vi "Page_Source_Send_To_MainDest_OnAdd.vi"(8 "error in (no error)":errorcluster, 11 "AB_Targetfile in":refnum<class "AB_Targetfile.lvclass">) -> (0 "error out":errorcluster, 2 "send to main dest":bool, 3 "AB_Targetfile out":refnum<class "AB_Targetfile.lvclass">)   [LabVIEW 2020, in "AB_Targetfile.lvclass"]
uses:
  <vilib>/AppBuilder/AB_Classes/TargetFile/AB_Targetfile.lvclass
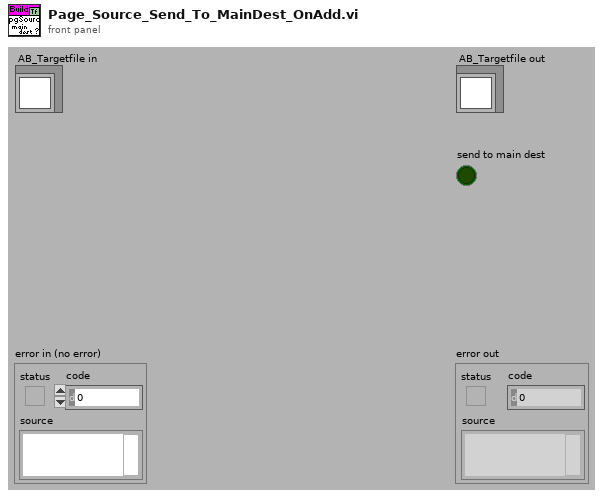
[diagram p1: front panel]
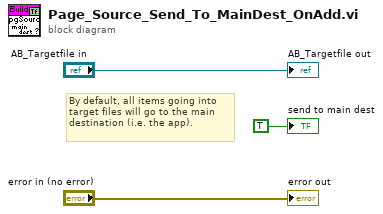
[diagram p0: block diagram]
diagram:
  # "By default, all items going into target files will go to the main destination (i.e. the app)."
  "error out" <- "error in (no error)"
  "AB_Targetfile out" <- "AB_Targetfile in"
  "send to main dest" <- TRUE ("send to main dest")
